vi "Delete Previous gRPC _server and _client Folder.vi"(8 "error in":errorcluster caption="error out", 10 "gRPC Service Name":string, 11 "PluginGenerator_MetaDataObj":refnum<class "PluginGenerator_MetaDataObj.lvclass">) -> (0 "error out":errorcluster, 3 "PluginGenerator_MetaDataObj out":refnum<class "PluginGenerator_MetaDataObj.lvclass">)   [LabVIEW 2021, in "Plugin Generator.lvlib"]
uses:
  Plugin Generator.lvlib
  PluginGenerator_MetaDataObj/PluginGenerator_MetaDataObj.lvclass
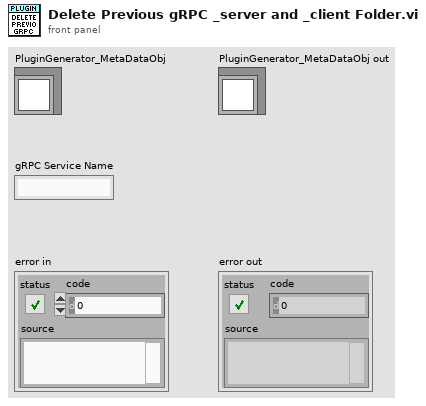
[diagram p1: front panel]
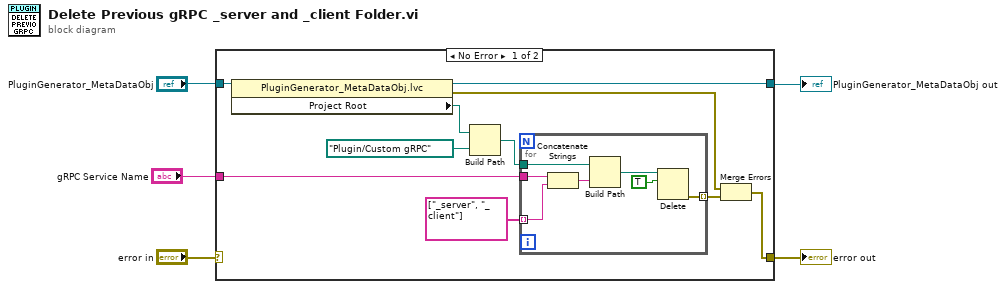
[diagram p0: block diagram]
diagram:
  n1 = case shown="No Error" "error in" {
    selector: "error in" -> [_ w24]
    tunnel: [w8 w24] -> w4
    tunnel: "PluginGenerator_MetaDataObj" -> [w12 w23]
    tunnel: [w7 w23] -> w2
    tunnel: "gRPC Service Name" -> [w6 _]
    frame No Error {
      n2 = property class="PluginGenerator_MetaDataObj.lvc"(reference=w12) -> (reference out=w7:refnum<class "PluginGenerator_MetaDataObj.lvclass">, error out=w9:errorcluster, "Project Root"=w11:path)  [unwired: 1 in]
      n3 = Build Path(base path=w11, name or relative path=path "Plugin/Custom gRPC") -> (appended path=w13:path)
      n4 = for {
        tunnel: [w22] -> w10 mode=indexing
        tunnel: w13 -> [w20]
        tunnel: w6 -> [w18]
        tunnel: string[] ["_server", "_client"] -> [w17] mode=indexing
        n5 = Concatenate Strings(w18, w17) -> (w19:string)
        n6 = Build Path(base path=w20, name or relative path=w19) -> (appended path=w16:path)
        n7 = Delete(path (use dialog)=w16, entire hierarchy (F)=TRUE) -> (error out=w22:errorcluster)  [unwired: 3 in, 2 out]
      }
      n8 = Merge Errors(w9, w10) -> (w8:errorcluster)
    }
    frame Error {
    }
  }
  "error out" <- w4
  "PluginGenerator_MetaDataObj out" <- w2
